vi "Configure.vi"(0 "File Actor in":refnum<class "File Actor.lvclass">) -> (14 "File Actor out":refnum<class "File Actor.lvclass">, 19 "error out":errorcluster)   [LabVIEW 2014, in "File Library.lvlib" / "File Actor.lvclass"]
uses:
  File Actor.lvclass
  reusable/Session APIs/File Access/Config Data/Config Data.lvclass
  Messages/To/Save/Change File Writing State MSG.lvclass
  <vilib>/ActorFramework/Actor/Actor.lvclass/Actor.ctl
  <vilib>/ActorFramework/Message Enqueuer/Message Enqueuer.lvclass/Message Enqueuer.ctl
  File Actor.lvclass/File Actor.ctl
  SuperActor/Ex Nested.lvclass/Ex Nested.ctl
  reusable/Session APIs/File Access/Config Data/Config Data.lvclass/Config Data.ctl
  Messages/To/Save/Change File Writing State MSG.lvclass/Change File Writing State MSG.ctl
  Read Cfg Header.vi
  SuperActor/Read ID.vi
  reusable/Session APIs/File Access/Config Data/Accessors/Read Ref.vi
  Messages/To/Save/Write Save_.vi
  <vilib>/ActorFramework/Message Enqueuer/Init from Existing Queue.vi
  <vilib>/Utility/config.llb/Read Key (String).vi
  <vilib>/Utility/config.llb/Read Key (Boolean).vi
  <vilib>/Utility/config.llb/Read Key (I32).vi
  <vilib>/ActorFramework/Message Priority Queue/Priority Enqueue.vi
  <vilib>/ActorFramework/Message Enqueuer/Message Enqueuer.lvclass
  <vilib>/Utility/config.llb/NI_LVConfig.lvlib
  <userlib>/_Session Fwk/Session - Root.lvclass
  <vilib>/ActorFramework/Actor/Actor.lvclass
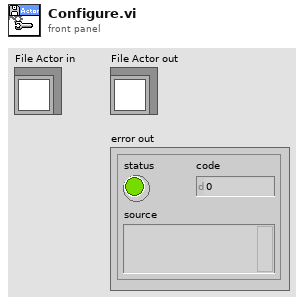
[diagram p1: front panel]
types:
  T1 = typedef "Session - Root.lvclass/Session Handle.ctl" = refnum<data-value>
  T2 = typedef "NI_LVConfig.lvlib/Config Data RefNum.ctl" = refnum<k1>
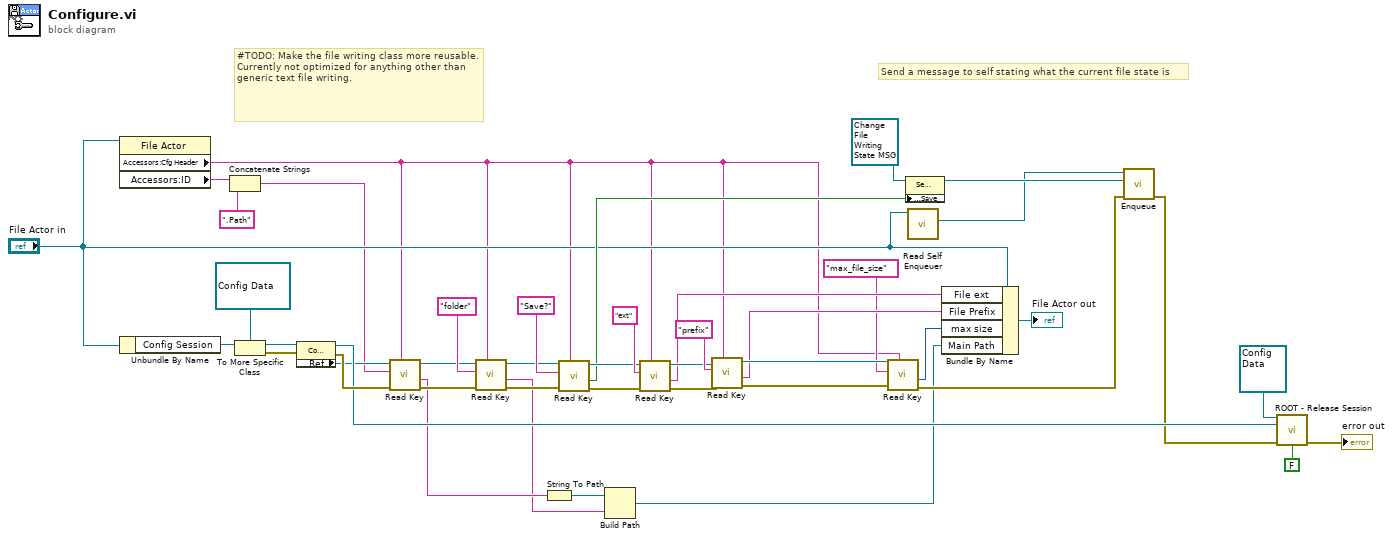
[diagram p0: block diagram]
diagram:
  # "Send a message to self stating what the current file state is"
  # "#TODO: Make the file writing class more reusable.  Currently not optimized for anything other than generic text file writing."
  n1 = property class="File Actor"(reference="File Actor in") -> ("Accessors:Cfg Header"=w9:string, "Accessors:ID"=w6:string)  [unwired: 1 in, 2 out]
  n2 = Unbundle By Name("File Actor in") -> ("Config Session"=w19:T1)
  n3 = Concatenate Strings(w6, ".Path" ("string")) -> (w7:string)
  n4 = To More Specific Class(target class=refnum<data-value> refnum ("Config Session"), reference=w19) -> (specific class reference=w20:refnum<data-value>, error out=w21:errorcluster)  [unwired: 1 in]
  n5 = property class="Config Data"(reference=w20, error in=w21) -> (reference out=w39:refnum<data-value>, error out=w42:errorcluster, "Accessors:Ref"=w22:T2)
  n6 = call-poly <vilib>:"Read Key.vi"("section"=w9, "error in (no error)"=w42, "key"=w7, "refnum"=w22) -> ("error out"=w24:errorcluster, "value"=w17:string, "refnum out"=w23:T2)  [unwired: 4 in, 1 out]
  n7 = call-poly <vilib>:"Read Key.vi"("section"=w9, "error in (no error)"=w24, "key"="folder", "refnum"=w23) -> ("error out"=w27:errorcluster, "value"=w12:string, "refnum out"=w26:T2)  [unwired: 4 in, 1 out]
  n8 = String To Path(string=w17) -> (path=w11:path)
  n9 = call-poly <vilib>:"Read Key.vi"("section"=w9, "error in (no error)"=w27, "key"="Save?", "refnum"=w26) -> ("error out"=w30:errorcluster, "value"=w16:bool, "refnum out"=w29:T2)  [unwired: 4 in, 1 out]
  n10 = Build Path(base path=w11, name or relative path=w12) -> (appended path=w1:path)
  n11 = call-poly <vilib>:"Read Key.vi"("section"=w9, "error in (no error)"=w30, "key"="ext", "refnum"=w29) -> ("error out"=w34:errorcluster, "value"=w32:string, "refnum out"=w33:T2)  [unwired: 4 in, 1 out]
  n12 = call-poly <vilib>:"Read Key.vi"("section"=w9, "error in (no error)"=w34, "key"="prefix", "refnum"=w33) -> ("error out"=w38:errorcluster, "value"=w36:string, "refnum out"=w37:T2)  [unwired: 4 in, 1 out]
  n13 = call-poly <vilib>:"Read Key.vi"("section"=w9, "error in (no error)"=w38, "key"="max_file_size", "refnum"=w37) -> ("error out"=w5:errorcluster, "value"=w13:i32)  [unwired: 4 in, 2 out]
  n14 = property class="Set File Save State"(reference=refnum<class "Change File Writing State MSG.lvclass"> refnum ("File Library.lvlib:Set File Save State"), "Accessors:Save_"=w16) -> (reference out=w3:refnum<class "Change File Writing State MSG.lvclass">)  [unwired: 1 in, 1 out]
  n15 = call <vilib>:"Read Self Enqueuer.vi"("Actor"="File Actor in") -> ("Self Enqueuer"=w2:refnum<class "Message Enqueuer.lvclass">)  [unwired: 10 in]
  n16 = Bundle By Name(cluster="File Actor in", "File ext"=w32, "File Prefix"=w36, "max size"=w13, "Main Path"=w1) -> (→"File Actor out":refnum<class "File Actor.lvclass">)
  n17 = call <vilib>:"Enqueue.vi"("error in (no error)"=w5, "Message"=w3, "Message Enqueuer in"=w2) -> ("error out"=w15:errorcluster)  [unwired: 7 in, 1 out]
  n18 = call <userlib>:"ROOT - Release Session.vi"("OBJ - Session in"=refnum<class "Config Data.lvclass"> refnum ("Config Data"), "Session Handle in"=w39, "error in (no error)"=w15, "force destroy? (F)"=FALSE) -> ("error out"=→"error out":errorcluster)  [unwired: 10 in, 1 out]
